vi "AddError.vi"(6 "NoErrorMessage":string="Vac OK", 7 "ErrorMessage":string="Unexpectced vacuum state. There might be a leak.", 8 "error in":errorcluster, 10 "code":i32=-999, 11 "Error?":bool) -> (0 "Error out":errorcluster)   [LabVIEW 2019]
uses:
  <vilib>/Utility/error.llb/DialogType.ctl
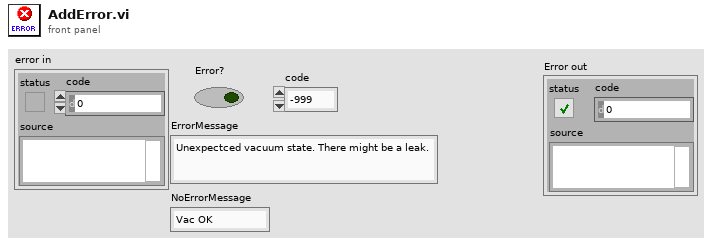
[diagram p1: front panel]
types:
  T1 = typedef "DialogType.ctl" = u16
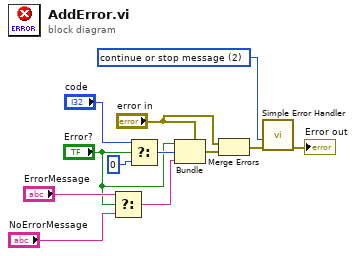
[diagram p0: block diagram]
diagram:
  w2 = T1 2 items=["no dialog", "OK message", "continue or stop message", "OK message + warnings", "continue/stop + warnings"] ("type of dialog (OK msg:1)")
  n1 = Select(t="ErrorMessage", s="Error?", f="NoErrorMessage") -> (s? t:f=w10:string)
  n2 = Select(t="code", s="Error?", f=0) -> (s? t:f=w7:i32)
  n3 = Bundle(cluster="error in", "status"="Error?", "code"=w7, "source"=w10) -> (w4:errorcluster)
  n4 = Merge Errors("error in", w4) -> (w3:errorcluster)
  n5 = call <vilib>:"Simple Error Handler.vi"("type of dialog (OK msg:1)"=w2, "error in (no error)"=w3) -> ("error out"=→"Error out":errorcluster)  [unwired: 3 in, 4 out]
